vi "Header or Footer.vi"(0 "OverContent":refnum<k24>, 2 "Header or Footer":T1, 5 "NumberOfPages":i32=1, 7 "pageNum":i32=1, 9 "Header or Footer Complete Cluster":T2, 11 "error in (no error)":errorcluster) -> (4 "OverContent duplicate":refnum<k24>, 15 "error out":errorcluster)   [LabVIEW 2019, in "Exaprom PDF.lvlib"]
doc: "Version 1.0\nDeveloped by Jean-Marc Simard\nCopyright © 2010, Exaprom Inc.\nAll rights reserved.\nLicense: BSD\n\nWith iTextSharp 4.1.6 (http://itextsharp.sourceforge.net)\nunder Mozilla Public License Version 1.1\n(http://www.mozilla.org/MPL/MPL-1.1.html)"
uses:
  C:/work/niobrara_lv/labview pdf writer fixing/DLL/itextsharp.dll
  DLL/itextsharp.dll
  Controls/Header, Footer and Watermark Controls/Header Footer Complete Cluster.ctl
  Controls/Header, Footer and Watermark Controls/Header or Footer Position.ctl
  Controls/Header, Footer and Watermark Controls/Header Footer Cluster with references.ctl
  Controls/Header, Footer and Watermark Controls/Header Footer Type.ctl
  Controls/Header, Footer and Watermark Controls/Header footer horiz alignment.ctl
  Controls/Table Controls/Cell Vertical alignment.ctl
  Controls/Header, Footer and Watermark Controls/Page number.ctl
  Controls/Font Controls/Font complete cluster horizontal.ctl
  Controls/Font Controls/Font size.ctl
  Controls/Font Controls/Font color.ctl
  Controls/Font Controls/Type and encoding.ctl
  Controls/Text Controls/Unicode/Type and run direction.ctl
  Controls/Header, Footer and Watermark Controls/Header Footer Line.ctl
  Controls/Text Controls/Line spacing.ctl
  Controls/Header, Footer and Watermark Controls/Header or Footer.ctl
  Exaprom PDF.lvlib
panel:
  # "X"
  # "Y"
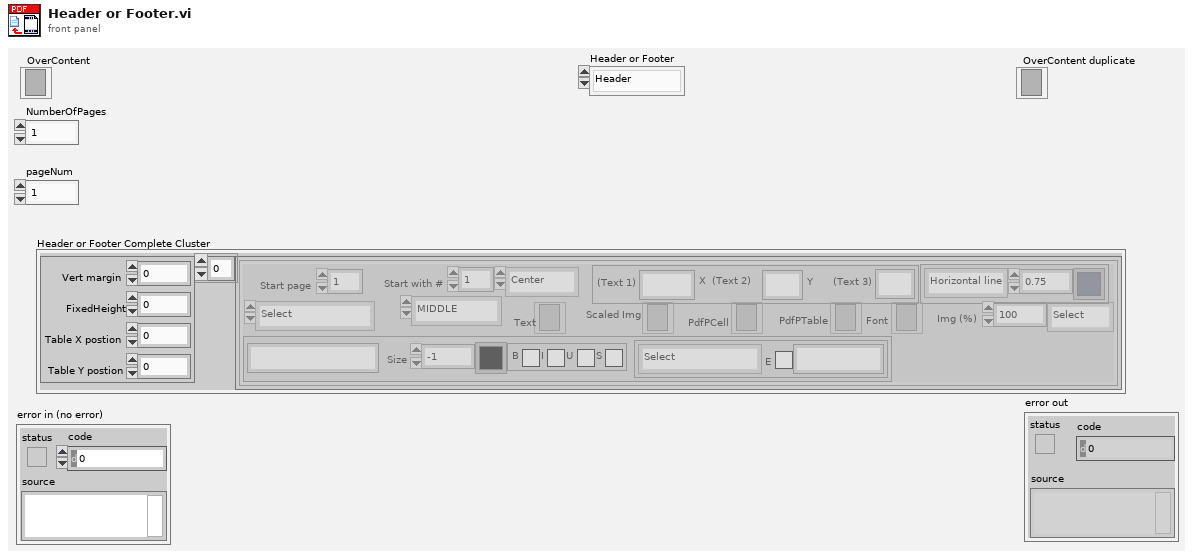
[diagram p1: front panel]
types:
  T1 = typedef "Exaprom PDF.lvlib/Header or Footer.ctl" = enum16{"Header", "Footer"}
  T2 = typedef "Exaprom PDF.lvlib/Header Footer Complete Cluster.ctl" = cluster{"Table position":T3, "Header Footer Cluster with references [ ]":T4[]}
  T3 = typedef "Exaprom PDF.lvlib/Header or Footer Position.ctl" = cluster{"Vert margin":dbl, "FixedHeight":dbl, "Table X postion":dbl, "Table Y postion":dbl}
  T4 = typedef "Exaprom PDF.lvlib/Header Footer Cluster with references.ctl" = cluster{"Start page":i32, "Type":T5, "Start with #":i32, "Alignment":T6, "Vertical Alignement":T7, "Page #":T8, "Text":refnum<k24>, "Scaled Img":refnum<k24>, "PdfPCell":refnum<k24>, "PdfPTable":refnum<k24>, "Font Cluster":T9, "Font ":refnum<k24>, "Img (%)":sgl, "Line":cluster{"Line":T14, "Thickness (points)":sgl, "Colour":T11}, "Line spacing":T15}
  T5 = typedef "Exaprom PDF.lvlib/Header Footer Type.ctl" = enum16{"Select", "Text", "Text + hyperlink", "Page number", "Image", "Image + hyperlink"}
  T6 = typedef "Exaprom PDF.lvlib/Header footer horiz alignment.ctl" = enum16{"Left", "Center", "Right"}
  T7 = typedef "Exaprom PDF.lvlib/Cell Vertical alignment.ctl" = enum16{"TOP", "MIDDLE", "BOTTOM"}
  T8 = typedef "Exaprom PDF.lvlib/Page number.ctl" = cluster{"Text 1":string, "Text 2":string, "Text 3":string}
  T9 = typedef "Exaprom PDF.lvlib/Font complete cluster horizontal.ctl" = cluster{"Name":string, "Size":T10, "Color":T11, "Style":cluster{"Bold":bool, "Italic":bool, "Underline":bool, "Strikeout":bool}, "Type":T12}
  T10 = typedef "Exaprom PDF.lvlib/Font size.ctl" = sgl
  T11 = typedef "Exaprom PDF.lvlib/Font color.ctl" = u32
  T12 = typedef "Exaprom PDF.lvlib/Type and encoding.ctl" = cluster{"Type&direction":T13, "Embedded":bool, "Encoding":string}
  T13 = typedef "Exaprom PDF.lvlib/Type and run direction.ctl" = enum16{"Select", "ASCII", "UTF-16", "UTF-16 (default)", "UTF-16 (LTR)", "UTF-16 (RTL)"}
  T14 = typedef "Exaprom PDF.lvlib/Header Footer Line.ctl" = enum16{"No line", "Horizontal line"}
  T15 = typedef "Exaprom PDF.lvlib/Line spacing.ctl" = enum16{"Select", "1.0", "1.5", "2.0"}
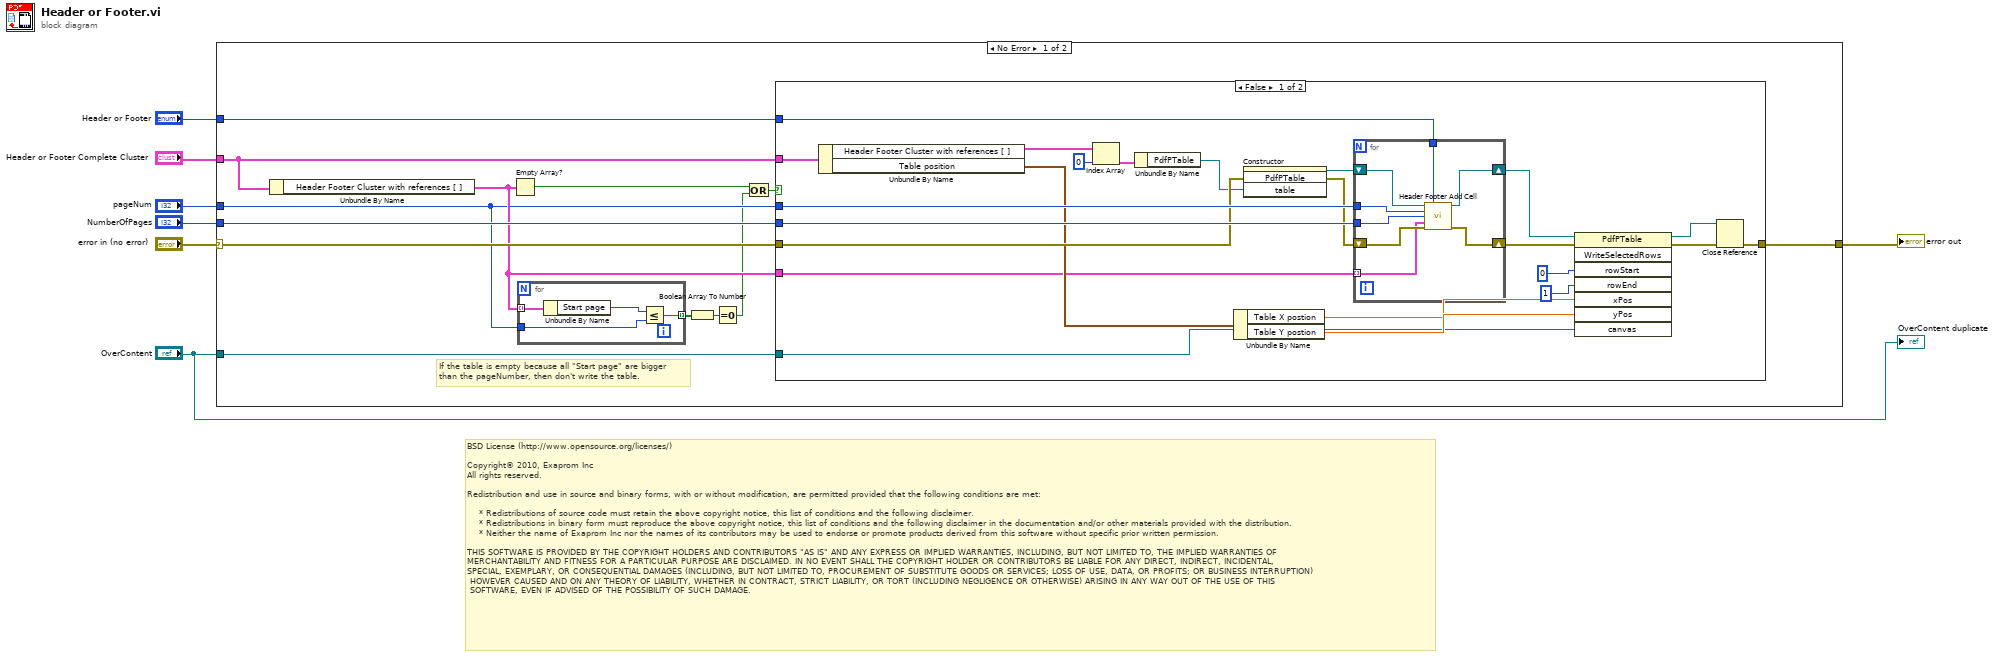
[diagram p0: block diagram]
diagram:
  # "BSD License (http://www.opensource.org/licenses/)\n\nCopyright© 2010, Exaprom Inc\nAll rights reserved.\n\nRedistribution and use in source and binary forms, with or without modification, are permitted provided that the following conditions are met:\n\n    * Redistributions of source code must retain the above copyright notice, this list of conditions and the following disclaimer.\n    * Redistributions in binary form must reproduce the above copyright notice, this list of conditions and the following disclaimer in the documentation and/or other materials provided with the distribution.\n    * Neither the name of Exaprom Inc nor the names of its contributors may be used to endorse or promote products derived from this software without specific prior written permission.\n\nTHIS SOFTWARE IS PROVIDED BY THE COPYRIGHT HOLDERS AND CONTRIBUTORS \"AS IS\" AND ANY EXPRESS OR IMPLIED WARRANTIES, INCLUDING, BUT NOT LIMITED TO, THE IMPLIED WARRANTIES OF \nMERCHANTABILITY AND FITNESS FOR A PARTICULAR PURPOSE ARE DISCLAIMED. IN NO EVENT SHALL THE COPYRIGHT HOLDER OR CONTRIBUTORS BE LIABLE FOR ANY DIRECT, INDIRECT, INCIDENTAL,\nSPECIAL, EXEMPLARY, OR CONSEQUENTIAL DAMAGES (INCLUDING, BUT NOT LIMITED TO, PROCUREMENT OF SUBSTITUTE GOODS OR SERVICES; LOSS OF USE, DATA, OR PROFITS; OR BUSINESS INTERRUPTION)\n HOWEVER CAUSED AND ON ANY THEORY OF LIABILITY, WHETHER IN CONTRACT, STRICT LIABILITY, OR TORT (INCLUDING NEGLIGENCE OR OTHERWISE) ARISING IN ANY WAY OUT OF THE USE OF THIS\n SOFTWARE, EVEN IF ADVISED OF THE POSSIBILITY OF SUCH DAMAGE."
  n1 = case shown="No Error" "error in (no error)" {
    selector: "error in (no error)" -> [w19 w57]
    tunnel: [w20 w57] -> w7
    tunnel: "pageNum" -> [w12 _]
    tunnel: "OverContent" -> [w18 _]
    tunnel: "NumberOfPages" -> [w17 _]
    tunnel: "Header or Footer Complete Cluster" -> [w16 _]
    tunnel: "Header or Footer" -> [w15 _]
    frame No Error {
      # "If the table is empty because all \"Start page\" are bigger\nthan the pageNumber, then don't write the table."
      n2 = Unbundle By Name(w16) -> ("Header Footer Cluster with references [ ]"=w13:T4[])
      n3 = Empty Array?(array=w13) -> (empty?=w9:bool)
      n4 = for {
        tunnel: w13 -> [w24] mode=indexing
        tunnel: w12 -> [w22]
        tunnel: [w21] -> w14 mode=indexing
        n5 = Unbundle By Name(w24) -> ("Start page"=w23:i32)
        n6 = Less Or Equal?(x=w23, y=w22) -> (x <= y?=w21:bool)
      }
      n7 = Boolean Array To Number(Boolean array=w14) -> (number=w11:u32)
      n8 = Equal To 0?(x=w11) -> (x = 0?=w8:bool)
      n9 = Or(x=w9, y=w8) -> (x .or. y?=w10:bool)
      n10 = case shown="False" w10 {
        tunnel: w12 -> [w44 _]
        tunnel: [w35 w56] -> w20
        tunnel: w19 -> [w39 w56]
        tunnel: w18 -> [w41 _]
        tunnel: w17 -> [w40 _]
        tunnel: w16 -> [w34 _]
        tunnel: w13 -> [w32 _]
        tunnel: w15 -> [w30 _]
        frame False {
          n11 = Unbundle By Name(w34) -> ("Header Footer Cluster with references [ ]"=w29:T4[], "Table position"=w33:T3)
          n12 = Index Array(array=w29, index=0) -> (element=w27:T4)
          n13 = Unbundle By Name(w27) -> ("PdfPTable"=w26:refnum<k24>)
          n14 = Unbundle By Name(w33) -> ("Table X postion"=w42:dbl, "Table Y postion"=w43:dbl)
          n15 = constructor class="PdfPTable"(error in=w39, "table"=w26) -> (reference out=w25:refnum<k24>, error out=w38:errorcluster)  [unwired: 2 in, 2 out]
          n16 = for {
            shift-right: [w52] -> w31
            shift-left: w25 -> [w53]
            shift-right: [w51] -> w45
            shift-left: w38 -> [w55]
            tunnel: w32 -> [w49] mode=indexing
            tunnel: w44 -> [w54]
            tunnel: w40 -> [w50]
            tunnel: w30 -> [w48]
            n17 = call "Header Footer Add Cell.vi"("PdfP Table"=w53, "Header or Footer"=w48, "Page #"=w54, "Total page #"=w50, "Header Footer Cluster with references"=w49, "error in (no error)"=w55) -> ("PdfP Table duplicate"=w52:refnum<k24>, "error out"=w51:errorcluster)  [unwired: 4 in, 4 out]
          }
          n18 = invoke class="PdfPTable" method="WriteSelectedRows"(reference=w31, error in=w45, "rowStart"=0, "rowEnd"=1, "xPos"=w42, "yPos"=w43, "canvas"=w41) -> (reference out=w36:refnum<k24>, error out=w37:errorcluster)  [unwired: 1 in, 6 out]
          n19 = Close Reference(reference=w36, error in (no error)=w37) -> (error out=w35:errorcluster)
        }
        frame True {
        }
      }
    }
    frame Error {
    }
  }
  "error out" <- w7
  "OverContent duplicate" <- "OverContent"
